vi "Update Icons.vi"(8 "error in (no error)":errorcluster, 11 "QControl Creation in":refnum<class "QControl Creation.lvclass">) -> (0 "error out":errorcluster, 3 "QControl Creation (dup)":refnum<class "QControl Creation.lvclass">)   [LabVIEW 2019, in "QControl Creation.lvclass"]
doc: "<b> </b> <b> </b>\n©2016 Q Software Innovations, LLC (QSI)\nwritten by Quentin Alldredge\nproduced in LabVIEW 2015\n\nsupport@qsoftwareinnovations.com\nwww.qsoftwareinnovations.com\n\nAll rights reserved.\n\nRedistribution and use in source and binary forms, with or without modification, are permitted provided that the following conditions are met:\n\n * Redistributions of source code must retain the above copyright notice, this list of conditions and the following disclaimer.\n * Redistributions in binary form must reproduce the above copyright notice, this list of conditions and the following disclaimer in the documentation and/or other materials provided with the distribution.\n * Neither the name of Q Software Innovations, LLC. nor the names of its contributors may be used to endorse or promote products derived from this software without specific prior written permission.\n\nTHIS SOFTWARE IS PROVIDED BY THE COPYRIGHT HOLDERS AND CONTRIBUTORS \"AS IS\" AND ANY EXPRESS OR IMPLIED WARRANTIES, INCLUDING, BUT NOT LIMITED TO, THE IMPLIED WARRANTIES OF MERCHANTABILITY AND FITNESS FOR A PARTICULAR PURPOSE ARE DISCLAIMED. IN NO EVENT SHALL THE COPYRIGHT OWNER OR CONTRIBUTORS BE LIABLE FOR ANY DIRECT, INDIRECT, INCIDENTAL, SPECIAL, EXEMPLARY, OR CONSEQUENTIAL DAMAGES (INCLUDING, BUT NOT LIMITED TO, PROCUREMENT OF SUBSTITUTE GOODS OR SERVICES; LOSS OF USE, DATA, OR PROFITS; OR BUSINESS INTERRUPTION) HOWEVER CAUSED AND ON ANY THEORY OF LIABILITY, WHETHER IN CONTRACT, STRICT LIABILITY, OR TORT (INCLUDING NEGLIGENCE OR OTHERWISE) ARISING IN ANY WAY OUT OF THE USE OF THIS SOFTWARE, EVEN IF ADVISED OF THE POSSIBILITY OF SUCH DAMAGE."
uses:
  QControl Creation.lvclass
  QControl Creation.lvclass/QControl Creation.ctl
  <vilib>/Utility/error.llb/Error Cluster From Error Code.vi
  <vilib>/ErrorRing/Error Ring.xnode
  <vilib>/LabVIEW Icon API/LabVIEW Icon API.lvlib
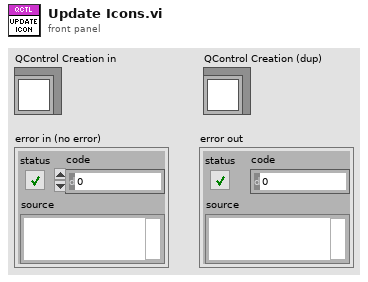
[diagram p1: front panel]
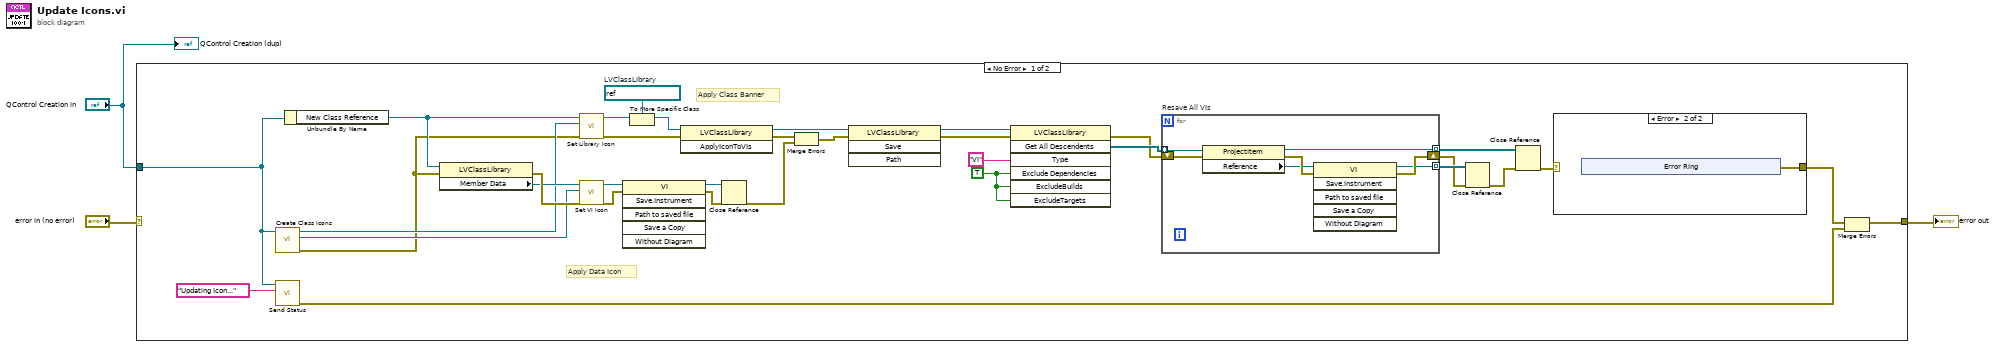
[diagram p0: block diagram]
diagram:
  n1 = case shown="No Error" "error in (no error)" {
    selector: "error in (no error)" -> [_ w52]
    tunnel: [w16 w52] -> w2
    tunnel: "QControl Creation in" -> [w17 _]
    frame No Error {
      w9 = refnum<vi> refnum  # LVClassLibrary
      w21 = TRUE ("ExcludeDependencies")
      # "Apply Data Icon"
      # "Apply Class Banner"
      n2 = call "Create Class Icons.vi"("QControl Creation in"=w17) -> ("error out"=w12:errorcluster, "Class Data Icon"=w23:refnum<class "Icon.lvclass">, "Class Banner Icon"=w24:refnum<class "Icon.lvclass">)  [unwired: 8 in]
      n3 = call "Send Status.vi"("Status"="Updating Icon..." ("Value"), "QControl Creation in"=w17) -> ("error out (dup)"=w15:errorcluster)  [unwired: 8 in, 1 out]
      n4 = Unbundle By Name(w17) -> ("New Class Reference"=w14:refnum<vi>)
      n5 = property class="LVClassLibrary"(reference=w14, error in=w12) -> (error out=w34:errorcluster, "Member Data"=w33:refnum<vi>)  [unwired: 1 out]
      n6 = call <vilib>:"Set Library Icon.vi"("error in (no error)"=w12, "Icon"=w24, "Library Refnum in"=w14) -> ("error out"=w8:errorcluster, "Library Refnum out"=w11:refnum<vi>)  [unwired: 7 in]
      n7 = call <vilib>:"Set VI Icon.vi"("error in (no error)"=w34, "Icon"=w23, "VI Refnum in"=w33) -> ("error out"=w36:errorcluster, "VI Refnum out"=w31:refnum<vi>)  [unwired: 7 in]
      n8 = invoke class="VI" method="Save.Instrument"(reference=w31, error in=w36) -> (reference out=w30:refnum<vi>, error out=w32:errorcluster)  [unwired: 4 in, 4 out]
      n9 = To More Specific Class(target class=w9, reference=w11) -> (specific class reference=w10:refnum<vi>)  [unwired: 1 in, 1 out]
      n10 = invoke class="LVClassLibrary" method="ApplyIconToVIs"(reference=w10, error in=w8) -> (reference out=w35:refnum<vi>, error out=w7:errorcluster)  [unwired: 1 in, 1 out]
      n11 = Close Reference(reference=w30, error in (no error)=w32) -> (error out=w6:errorcluster)
      n12 = Merge Errors(w7, w6) -> (w13:errorcluster)
      n13 = invoke class="LVClassLibrary" method="Save"(reference=w35, error in=w13) -> (reference out=w29:refnum<vi>, error out=w37:errorcluster)  [unwired: 2 in, 2 out]
      n14 = invoke class="LVClassLibrary" method="Get All Descendents"(reference=w29, error in=w37, "Type"="VI", "Exclude Dependencies"=w21, "ExcludeBuilds"=w21, "ExcludeTargets"=w21) -> (error out=w27:errorcluster, "All Descendents"=w28:refnum<vi>[])  [unwired: 1 in, 5 out]
      n15 = for "Resave All VIs" {
        tunnel: w28 -> [w48] mode=indexing
        tunnel: [w46] -> w26 mode=indexing
        shift-right: [w50] -> w25
        shift-left: w27 -> [w51]
        tunnel: [w45] -> w20 mode=indexing
        n16 = property class="ProjectItem"(reference=w48, error in=w51) -> (reference out=w45:refnum<vi>, error out=w49:errorcluster, "Reference"=w47:refnum<vi>)
        n17 = invoke class="VI" method="Save.Instrument"(reference=w47, error in=w49) -> (reference out=w46:refnum<vi>, error out=w50:errorcluster)  [unwired: 4 in, 4 out]
      }
      n18 = Close Reference(reference=w26, error in (no error)=w25) -> (error out=w19:errorcluster)
      n19 = Close Reference(reference=w20, error in (no error)=w19) -> (error out=w5:errorcluster)
      n20 = case shown="Error" w5 {
        selector: w5 -> [w38 _]
        tunnel: [w38 w39] -> w4
        frame No Error {
        }
        frame Error {
          n21 = xnode "Error Ring"() -> ("error out"=w39:errorcluster)
        }
      }
      n22 = Merge Errors(w4, w15) -> (w16:errorcluster)
    }
    frame Error {
    }
  }
  "error out" <- w2
  "QControl Creation (dup)" <- "QControl Creation in"
